vi "Construct Robots.vi"(1 "Total Steps to be Executed":i32, 2 "Factory Status":T4, 4 "Robot Building Costs":T1 {"Geode"."Mineral" items=["Ore", "Clay", "Obsidian", "Geode", "Open Geode"]; "Obsidian"."Mineral" items=["Ore", "Clay", "Obsidian", "Geode", "Open Geode"]; "Clay"."Mineral" items=["Ore", "Clay", "Obsidian", "Geode", "Open Geode"]; "Ore"."Mineral" items=["Ore", "Clay", "Obsidian", "Geode", "Open Geode"]}) -> (5 "Consumed Materials":T5, 6 "Constructed Robots":T6)   [LabVIEW 2020, in "AoC 2022.lvlib"]
uses:
  AoC 2022.lvlib
  Robot Factory.ctl
  Inventory.ctl
  Step.ctl
  Robot Building Costs.ctl
  Cost.ctl
  Mineral.ctl
  Mineral_Enum.ctl
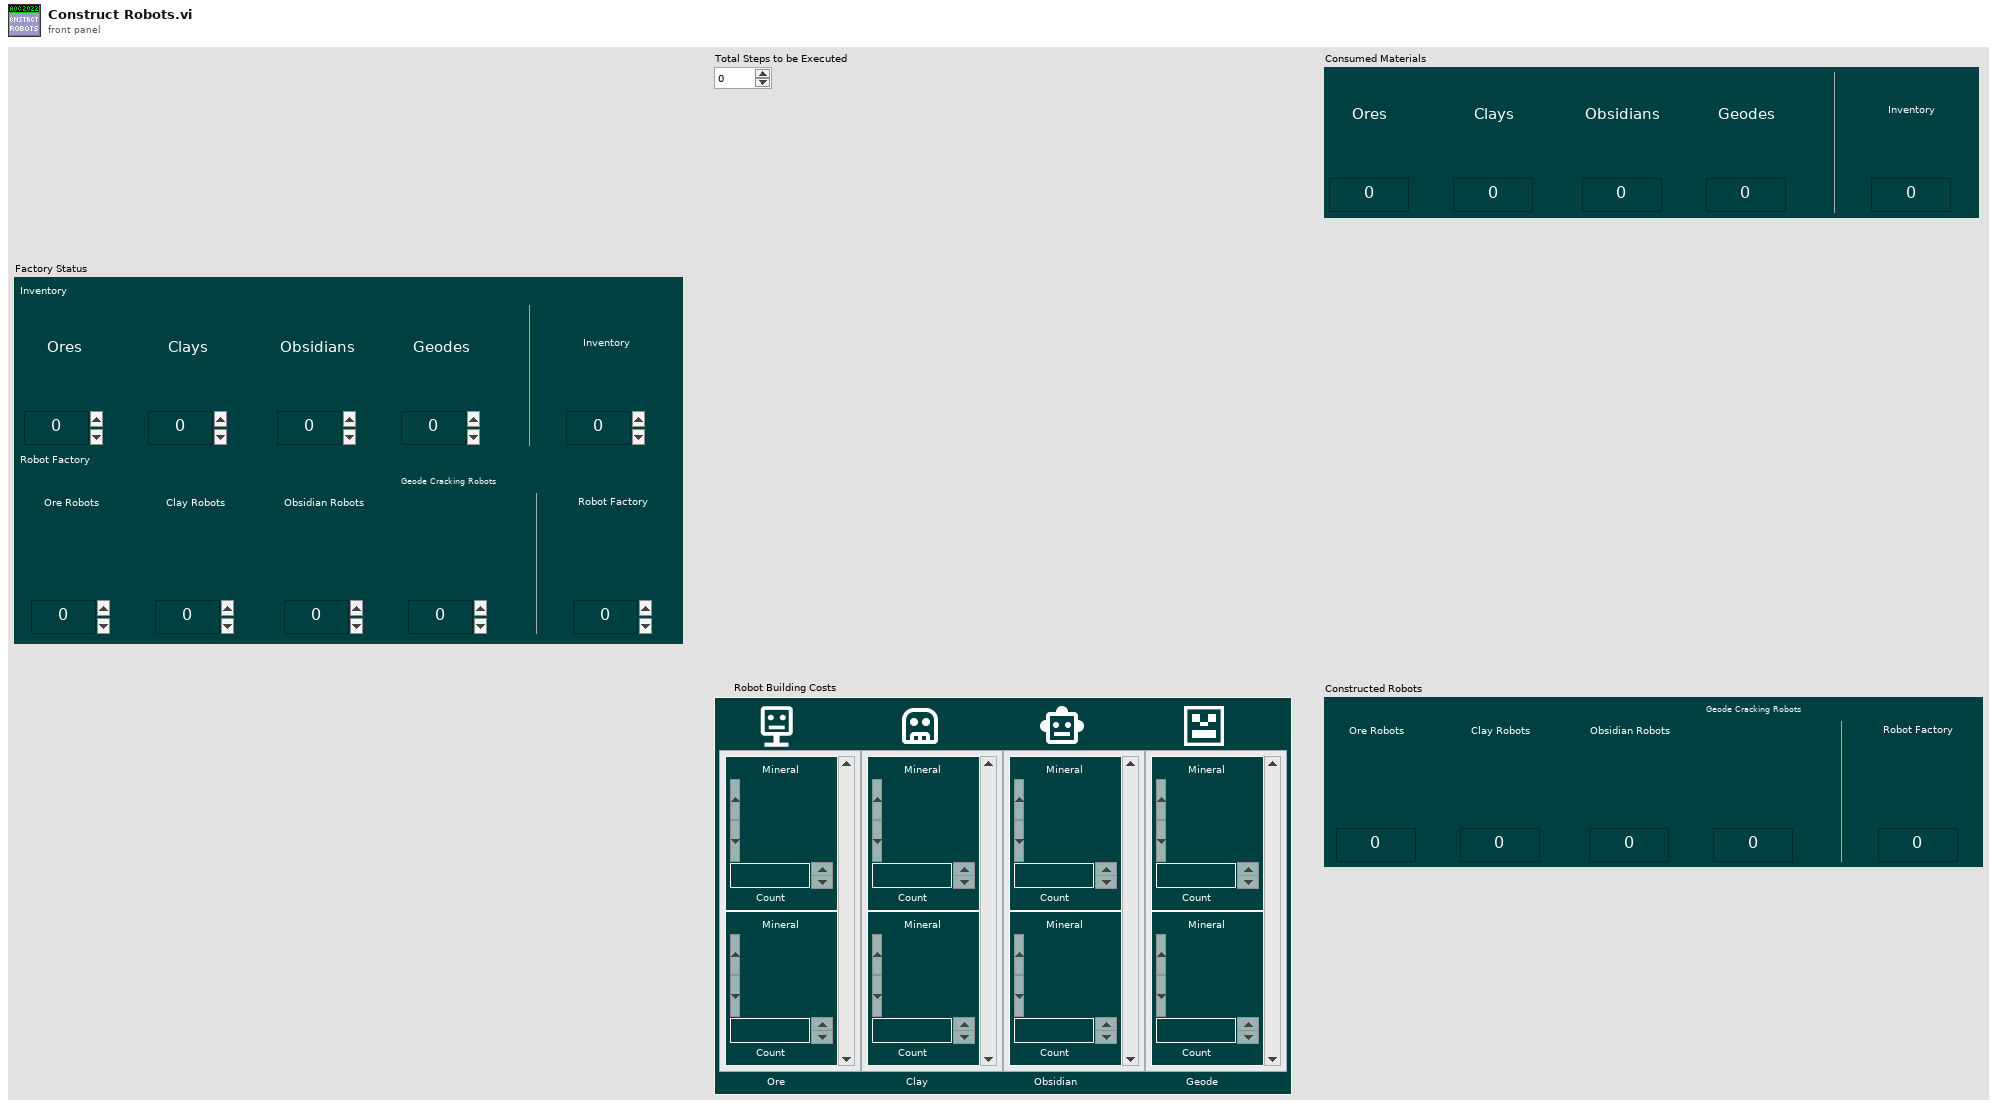
[diagram p1: front panel]
types:
  T1 = typedef "AoC 2022.lvlib/Robot Building Costs.ctl" = cluster{"Ore":T2[], "Clay":T2[], "Obsidian":T2[], "Geode":T2[]}
  T2 = typedef "AoC 2022.lvlib/Cost.ctl" = cluster{"Mineral":T3, "Count":u32}
  T3 = typedef "AoC 2022.lvlib/Mineral.ctl" = u16
  T4 = typedef "AoC 2022.lvlib/Step.ctl" = cluster{"Inventory":T5, "Robot Factory":T6}
  T5 = typedef "AoC 2022.lvlib/Inventory.ctl" = cluster{"Ores":u32, "Clays":u32, "Obsidians":u32, "Geodes":u32, "Inventory":u32}
  T6 = typedef "AoC 2022.lvlib/Robot Factory.ctl" = cluster{"Ore Robots":u32, "Clay Robots":u32, "Obsidian Robots":u32, "Geode Cracking Robots":u32, "Robot Factory":u32}
  T7 = typedef "AoC 2022.lvlib/Mineral_Enum.ctl" = enum16{"ore", "clay", "obsidian", "geode", "Open Geode"}
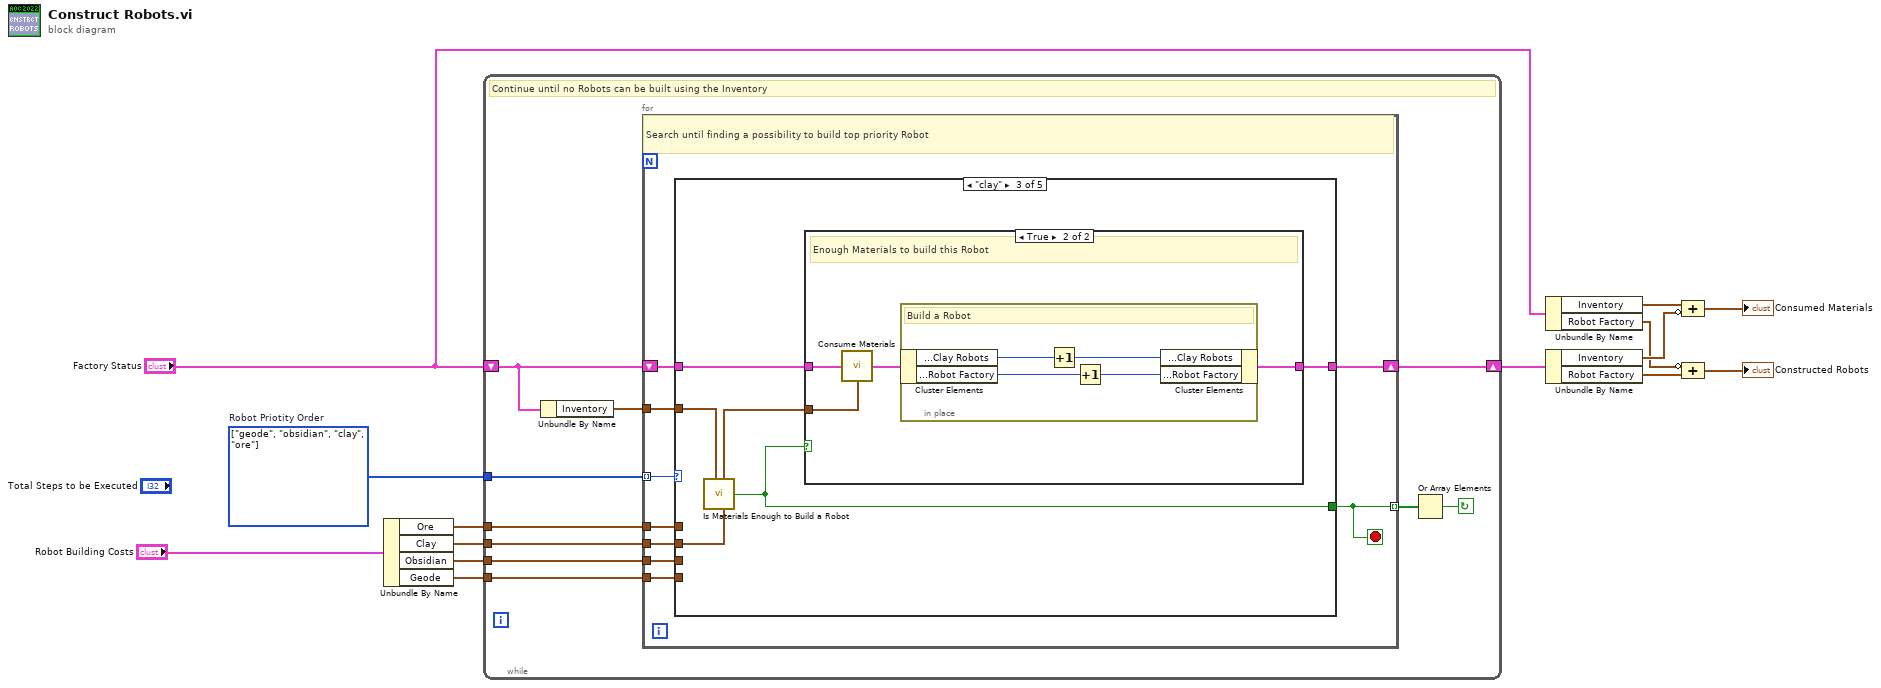
[diagram p0: block diagram]
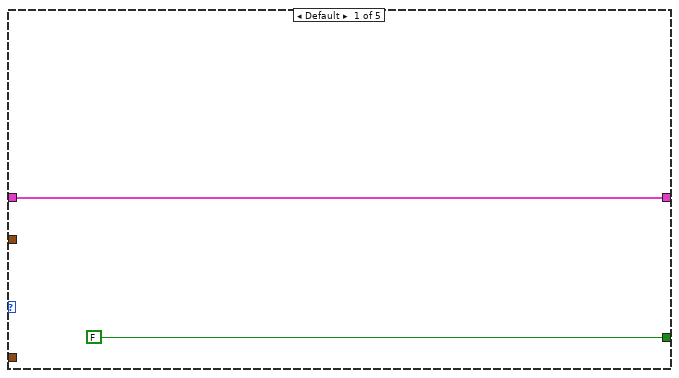
[diagram p2: hidden frame]
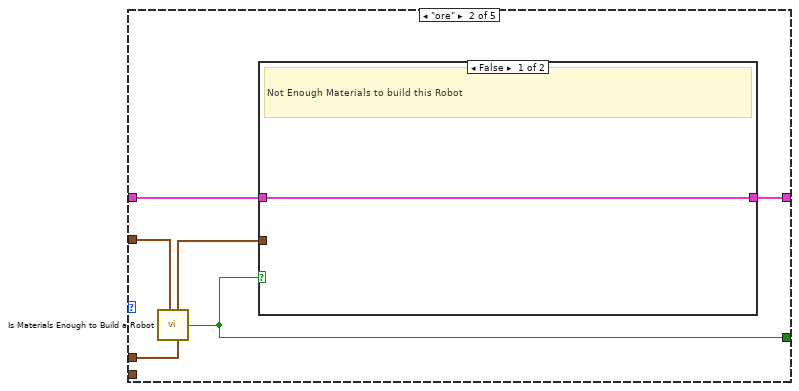
[diagram p3: hidden frame]
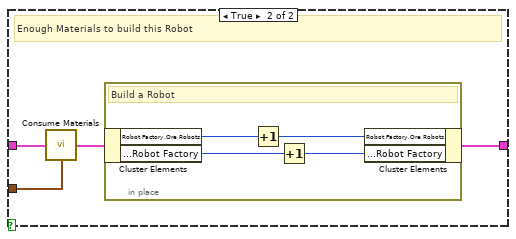
[diagram p4: hidden frame]
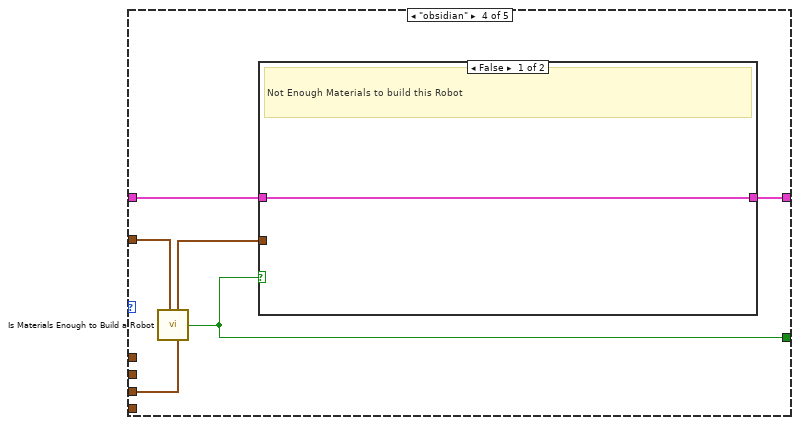
[diagram p6: hidden frame]
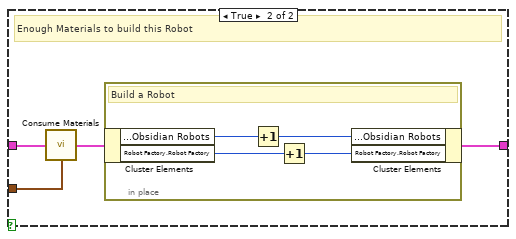
[diagram p7: hidden frame]
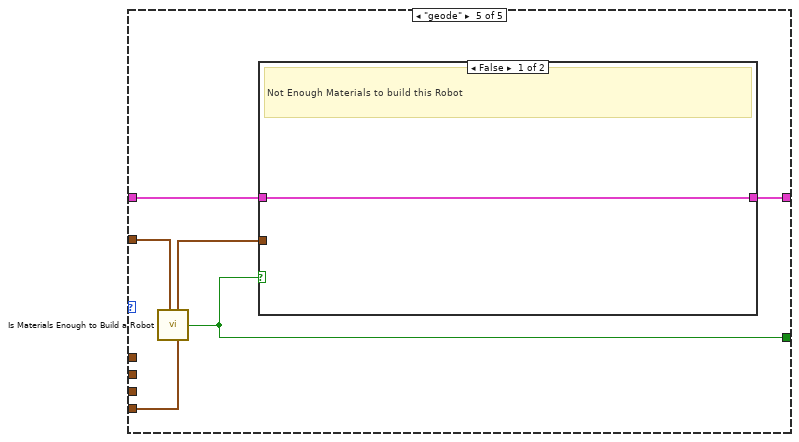
[diagram p8: hidden frame]
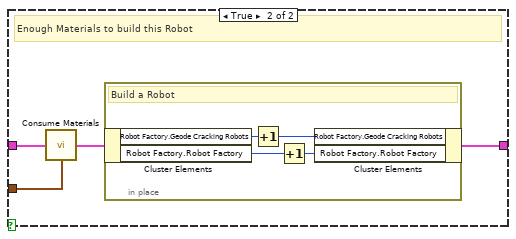
[diagram p9: hidden frame]
diagram:
  w14 = T7[] [enum."geode", enum."obsidian", enum."clay", enum."ore"] items=["ore", "clay", "obsidian", "geode", "Open Geode"]  # Robot Priotity Order
  n1 = Unbundle By Name("Robot Building Costs") -> ("Ore"=w12:T2[], "Clay"=w11:T2[], "Obsidian"=w10:T2[], "Geode"=w9:T2[])
  n2 = while {
    shift-right: [w24] -> w7
    shift-left: "Factory Status" -> [w16]
    tunnel: w14 -> [w23]
    tunnel: w12 -> [w20]
    tunnel: w11 -> [w19]
    tunnel: w10 -> [w18]
    tunnel: w9 -> [w17]
    stop <- w21 continue-if-true
    # "Continue until no Robots can be built using the Inventory"
    n3 = Unbundle By Name(w16) -> ("Inventory"=w15:T5)
    n4 = for {
      tunnel: w23 -> [w31] mode=indexing
      shift-right: [w33] -> w24
      shift-left: w16 -> [w32]
      tunnel: [w30] -> w22 mode=indexing
      tunnel: w20 -> [w29]
      tunnel: w19 -> [w28]
      tunnel: w18 -> [w27]
      tunnel: w17 -> [w26]
      tunnel: w15 -> [w25]
      stop <- w30 stop-if-true
      # "Search until finding a possibility to build top priority Robot"
      n5 = case shown="\"clay\"" w31 {
        tunnel: [w35 w39 w53 w67 w81] -> w33
        tunnel: w32 -> [w35 w38 w52 w66 w80]
        tunnel: [FALSE w40 w54 w68 w82] -> w30
        tunnel: w29 -> [_ w37 _ _ _]
        tunnel: w28 -> [_ _ w50 _ _]
        tunnel: w27 -> [_ _ _ w64 _]
        tunnel: w26 -> [_ _ _ _ w78]
        tunnel: w25 -> [_ w36 w51 w65 w79]
        frame Default {
        }
        frame "ore" {
          n6 = call "Is Materials Enough to Build a Robot.vi"("Inventory"=w36, "Robot Building Cost"=w37) -> ("Is Materials Enough to Build a Robot ?"=w40:bool)  [unwired: 1 in]
          n7 = case shown="False" w40 {
            tunnel: [w41 w43] -> w39
            tunnel: w38 -> [w41 w44]
            tunnel: w37 -> [_ w45]
            frame False {
              # "Not Enough Materials to build this Robot"
            }
            frame True {
              # "Enough Materials to build this Robot"
              n8 = call "Consume Materials.vi"("Factory Status in"=w44, "Materials"=w45) -> ("Factory Status out"=w42:T4)
              n9 = in-place {
                # "Build a Robot"
                n10 = in-place-cluster #1(w42) -> ("Robot Factory.Ore Robots"=w49:u32, "Robot Factory.Robot Factory"=w48:u32)
                n11 = Increment(x=w49) -> (x+1=w46:u32)
                n12 = Increment(x=w48) -> (x+1=w47:u32)
                n13 = in-place-cluster #1("Robot Factory.Ore Robots"=w46, "Robot Factory.Robot Factory"=w47) -> (w43:T4)
              }
            }
          }
        }
        frame "clay" {
          n14 = call "Is Materials Enough to Build a Robot.vi"("Inventory"=w51, "Robot Building Cost"=w50) -> ("Is Materials Enough to Build a Robot ?"=w54:bool)  [unwired: 1 in]
          n15 = case shown="True" w54 {
            tunnel: [w55 w57] -> w53
            tunnel: w52 -> [w55 w58]
            tunnel: w50 -> [_ w59]
            frame False {
              # "Not Enough Materials to build this Robot"
            }
            frame True {
              # "Enough Materials to build this Robot"
              n16 = call "Consume Materials.vi"("Factory Status in"=w58, "Materials"=w59) -> ("Factory Status out"=w56:T4)
              n17 = in-place {
                # "Build a Robot"
                n18 = in-place-cluster #2(w56) -> ("Robot Factory.Clay Robots"=w63:u32, "Robot Factory.Robot Factory"=w62:u32)
                n19 = Increment(x=w63) -> (x+1=w60:u32)
                n20 = Increment(x=w62) -> (x+1=w61:u32)
                n21 = in-place-cluster #2("Robot Factory.Clay Robots"=w60, "Robot Factory.Robot Factory"=w61) -> (w57:T4)
              }
            }
          }
        }
        frame "obsidian" {
          n22 = call "Is Materials Enough to Build a Robot.vi"("Inventory"=w65, "Robot Building Cost"=w64) -> ("Is Materials Enough to Build a Robot ?"=w68:bool)  [unwired: 1 in]
          n23 = case shown="False" w68 {
            tunnel: [w69 w71] -> w67
            tunnel: w66 -> [w69 w72]
            tunnel: w64 -> [_ w73]
            frame False {
              # "Not Enough Materials to build this Robot"
            }
            frame True {
              # "Enough Materials to build this Robot"
              n24 = call "Consume Materials.vi"("Factory Status in"=w72, "Materials"=w73) -> ("Factory Status out"=w70:T4)
              n25 = in-place {
                # "Build a Robot"
                n26 = in-place-cluster #3(w70) -> ("Robot Factory.Obsidian Robots"=w77:u32, "Robot Factory.Robot Factory"=w76:u32)
                n27 = Increment(x=w77) -> (x+1=w74:u32)
                n28 = Increment(x=w76) -> (x+1=w75:u32)
                n29 = in-place-cluster #3("Robot Factory.Obsidian Robots"=w74, "Robot Factory.Robot Factory"=w75) -> (w71:T4)
              }
            }
          }
        }
        frame "geode" {
          n30 = call "Is Materials Enough to Build a Robot.vi"("Inventory"=w79, "Robot Building Cost"=w78) -> ("Is Materials Enough to Build a Robot ?"=w82:bool)  [unwired: 1 in]
          n31 = case shown="False" w82 {
            tunnel: [w83 w85] -> w81
            tunnel: w80 -> [w83 w86]
            tunnel: w78 -> [_ w87]
            frame False {
              # "Not Enough Materials to build this Robot"
            }
            frame True {
              # "Enough Materials to build this Robot"
              n32 = call "Consume Materials.vi"("Factory Status in"=w86, "Materials"=w87) -> ("Factory Status out"=w84:T4)
              n33 = in-place {
                # "Build a Robot"
                n34 = in-place-cluster #4(w84) -> ("Robot Factory.Geode Cracking Robots"=w91:u32, "Robot Factory.Robot Factory"=w90:u32)
                n35 = Increment(x=w91) -> (x+1=w88:u32)
                n36 = Increment(x=w90) -> (x+1=w89:u32)
                n37 = in-place-cluster #4("Robot Factory.Geode Cracking Robots"=w88, "Robot Factory.Robot Factory"=w89) -> (w85:T4)
              }
            }
          }
        }
      }
    }
    n38 = Or Array Elements(Boolean array=w22) -> (logical OR=w21:bool)
  }
  n39 = Unbundle By Name("Factory Status") -> ("Inventory"=w6:T5, "Robot Factory"=w3:T6)
  n40 = Unbundle By Name(w7) -> ("Inventory"=w5:T5, "Robot Factory"=w2:T6)
  n41 = Compound Arithmetic op=ADD(w6, invert w5) -> (→"Consumed Materials":T5)
  n42 = Compound Arithmetic op=ADD(invert w3, w2) -> (→"Constructed Robots":T6)
